vi "Capture Analyzer Measurement Select Folder.vi"(8 "error in (no error)":errorcluster, 9 "Select Folder (\"folder\")":string="folder", 10 "Instance (1)":i32=1, 11 "VISA resource name":refnum<visa-resource-name>) -> (0 "error out":errorcluster, 3 "VISA resource name out":refnum<visa-resource-name>)   [LabVIEW 2020, in "Rohde&Schwarz CMXP GPRF.lvlib"]
doc: "Selects a folder for storage of all buffer contents to files (I/Q data for all segments).\nThe default folder is @USERDATA\\captureanalyzer. You can only select a subfolder of this default folder.\nAll files within the selected folder are deleted when the capture buffer analyzer writes the result files.\n\nAttribute:\nRSCMXPGPRF_ATTR_CAPTURE_ANALYZER_MEASUREMENT_STORAGE_FOLDER\n\nRemote-control command:\nCONFigure:GPRF:MEAS<i>:CANalyzer:SALL:IQFolder"
uses:
  <instrlib>/Rohde&Schwarz CMXP GPRF/Rohde&Schwarz CMXP GPRF.lvlib
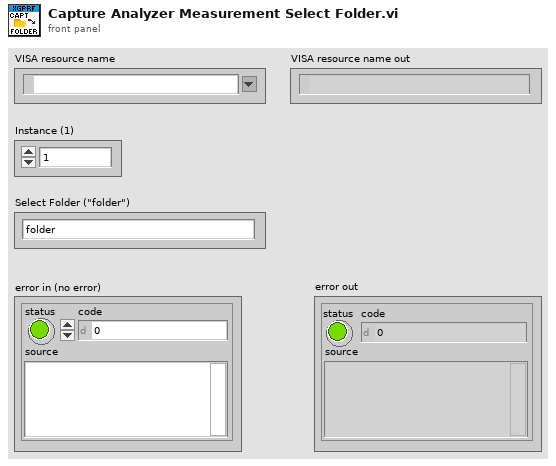
[diagram p1: front panel]
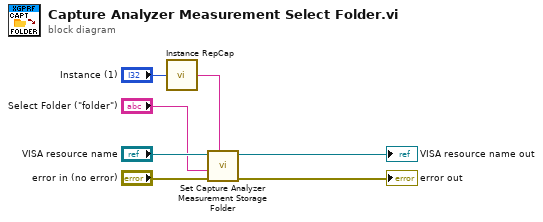
[diagram p0: block diagram]
diagram:
  n1 = call <instrlib>:"Instance RepCap.vi"("Instance in"="Instance (1)") -> ("Instance out"=w2:string)
  n2 = call "Set Capture Analyzer Measurement Storage Folder"("Repeated Capabilities"=w2, "error in (no error)"="error in (no error)", "Capture Analyzer Measurement Storage Folder ()"="Select Folder (\"folder\")", "instrument handle"="VISA resource name") -> ("error out"=→"error out":errorcluster, "instrument handle out"=→"VISA resource name out":refnum<visa-resource-name>)  [unwired: 6 in]
